vi "FragRlue.vi"() -> ()   [LabVIEW 2019]
uses:
  <vilib>/numeric/Random Number (Range) DBL.vi
panel:
  in  "inputSignal":bool
  out "GreenSignal":bool
  out "RedSignal":bool
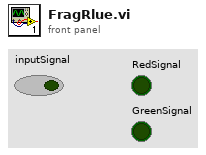
[diagram p1: front panel]
types:
  T1 = cluster{"InternalTimer":u32, "State":enum16{"Ready", "RedSignal", "OffSignal", "GreenSignal"}}
  T2 = enum16{"Ready", "RedSignal", "OffSignal", "GreenSignal"}
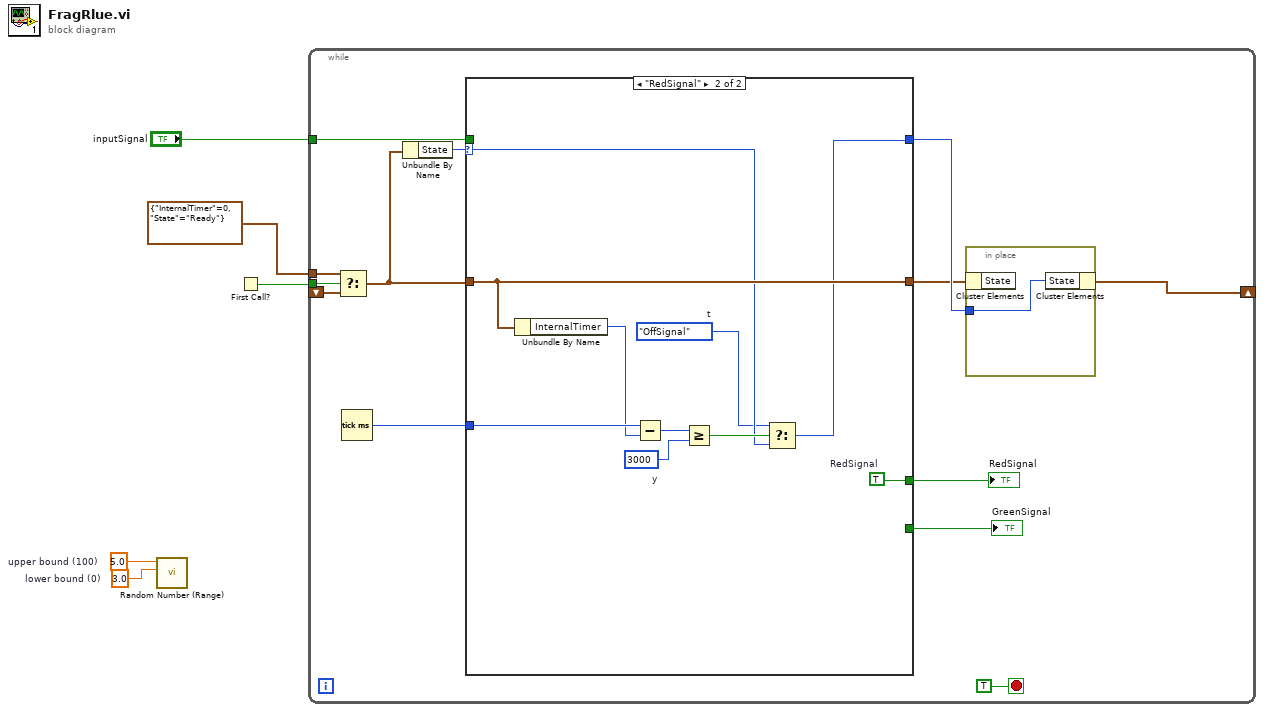
[diagram p0: block diagram]
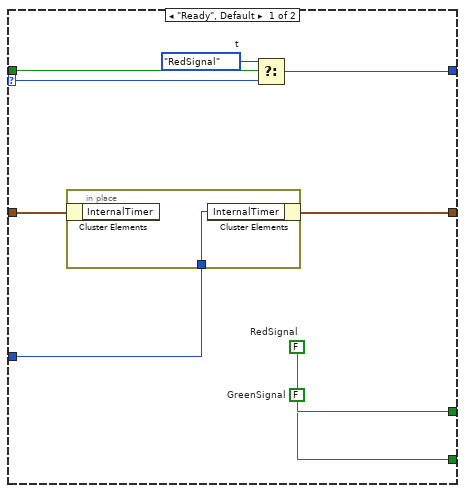
[diagram p2: hidden frame]
diagram:
  w4 = 5.0  # upper bound (100)
  w5 = 3.0  # lower bound (0)
  n1 = call-poly <vilib>:"Random Number (Range).vi"("lower bound (0)"=w5, "upper bound (100)"=w4) -> ()  [unwired: 9 in, 1 out]
  n2 = First Call?() -> (First Call?: T/F=w2:bool)
  n3 = while {
    tunnel: "inputSignal" -> [w17]
    shift-right: [w12] -> _
    shift-left: _ -> [w8]
    tunnel: w2 -> [w9]
    tunnel: T1 {"InternalTimer"=0, "State"=enum."Ready"} -> [w7]
    stop <- TRUE stop-if-true
    n4 = Select(t=w7, s=w9, f=w8) -> (s? t:f=w6:T1)
    n5 = Tick Count (ms)() -> (millisecond timer value=w10:u32)
    n6 = Unbundle By Name(w6) -> ("State"=w14:T2)
    n7 = case shown="\"RedSignal\"" w14 {
      selector: w14 -> [w27 w32]
      tunnel: w17 -> [w28 _]
      tunnel: [w25 w31] -> w13
      tunnel: [w24 w39] -> w16
      tunnel: [w23 _] -> w15
      tunnel: w6 -> [w22 w38]
      tunnel: [w21 w38] -> w11
      tunnel: w10 -> [w20 w37]
      frame "Ready", Default {
        w23 = FALSE  # GreenSignal
        w24 = FALSE  # RedSignal
        w26 = T2."RedSignal"  # t
        n8 = in-place {
          in-place-border: w20 -> [w29]
          n9 = in-place-cluster #1(w22) -> ()  [unwired: 1 out]
          n10 = in-place-cluster #1("InternalTimer"=w29) -> (w21:T1)
        }
        n11 = Select(t=w26, s=w28, f=w27) -> (s? t:f=w25:T2)
      }
      frame "RedSignal" {
        w30 = T2."OffSignal"  # t
        w34 = u32 3000  # y
        w39 = TRUE  # RedSignal
        n12 = Unbundle By Name(w38) -> ("InternalTimer"=w36:u32)
        n13 = Subtract(x=w37, y=w36) -> (x-y=w35:u32)
        n14 = Greater Or Equal?(x=w35, y=w34) -> (x >= y?=w33:bool)
        n15 = Select(t=w30, s=w33, f=w32) -> (s? t:f=w31:T2)
      }
    }
    "RedSignal" <- w16
    "GreenSignal" <- w15
    n16 = in-place {
      in-place-border: w13 -> [w19]
      n17 = in-place-cluster #2(w11) -> ()  [unwired: 1 out]
      n18 = in-place-cluster #2("State"=w19) -> (w12:T1)
    }
  }
